vi "GUI Init - AOM.vi"(7 "Disabled":T1(ring), 8 "error in (no error)":errorcluster, 9 "Ch.names":string[](array[string]), 10 "Cluster":T3 {"Ch.value" min=-10.0 max=20.0 step=1.0 format="%.3g"}, 11 "GUI Refs":T2) -> (0 "error out":errorcluster, 2 "Data":dbl[](array[numeric]), 3 "reference out":refnum<vi>)   [LabVIEW 2017]
doc: "Initialize array's size and values for AOM Array by reference"
uses:
  Controls/AOM_GUI_Cluster.ctl
  Controls/GUI Referencies.ctl
  Controls/TDMS_GUI_Cluster.ctl
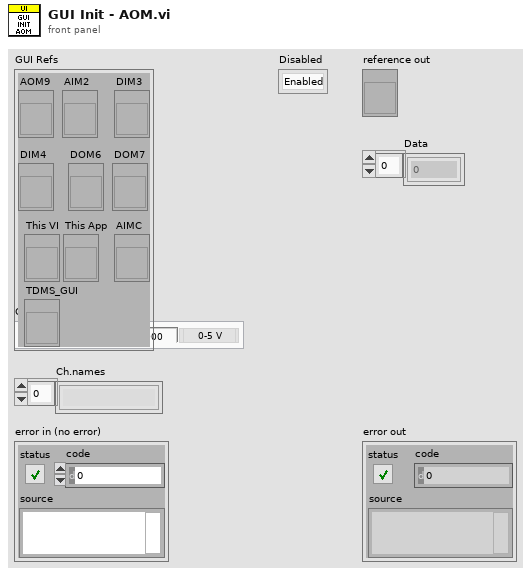
[diagram p1: front panel]
types:
  T1 = enum8{"Enabled", "Disabled", "Disabled and Grayed Out"}
  T2 = typedef "GUI Referencies.ctl" = cluster{"This VI":refnum<vi>, "This App":refnum<vi>, "DIM3":refnum<vi>, "DIM4":refnum<vi>, "DOM6":refnum<vi>, "DOM7":refnum<vi>, "AOM9":refnum<vi>, "AIM2":refnum<vi>, "AIMC":refnum<vi>, "TDMS_GUI":refnum<vi>}
  T3 = typedef "AOM_GUI_Cluster.ctl" = cluster{"Ch.name":string, "Ch.value":dbl, "Ch.mode":enum16{"0-5 V", "+/-10 V", "0-5 mA", "4-20 mA"}, "Num":string}
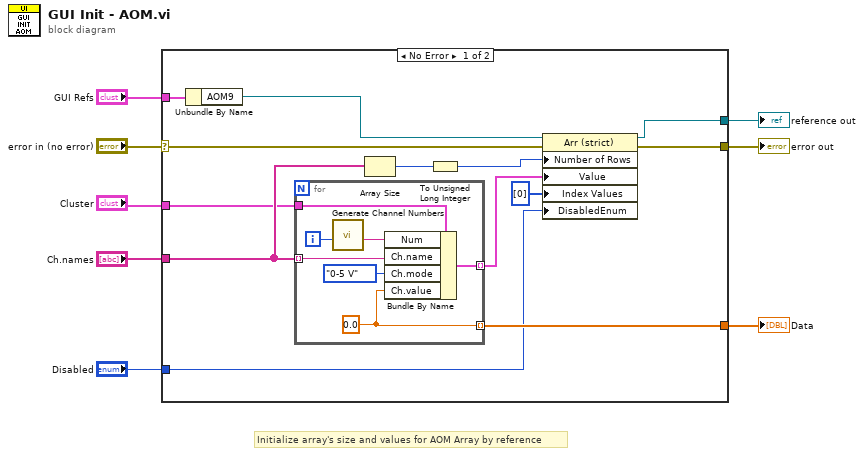
[diagram p0: block diagram]
diagram:
  # "Initialize array's size and values for AOM Array by reference"
  n1 = case shown="No Error" "error in (no error)" {
    selector: "error in (no error)" -> [w16 w29]
    tunnel: [w15 w29] -> w7
    tunnel: "Ch.names" -> [w18 _]
    tunnel: "GUI Refs" -> [w12 _]
    tunnel: "Cluster" -> [w17 _]
    tunnel: [w14 _] -> w4
    tunnel: [w10 _] -> w2
    tunnel: "Disabled" -> [w9 _]
    frame No Error {
      n2 = Unbundle By Name(w12) -> ("AOM9"=w11:refnum<vi>)
      n3 = for {
        tunnel: [w28] -> w14 mode=indexing
        tunnel: [w27] -> w13 mode=indexing
        tunnel: w18 -> [w26] mode=indexing
        tunnel: w17 -> [w25]
        i -> [w22]
        w28 = 0.0 ("Ch.value")
        n4 = call "Generate Channel Numbers.vi"("Index"=w22) -> ("Number"=w23:string)  [unwired: 9 in, 1 out]
        n5 = Bundle By Name(cluster=w25, "Num"=w23, "Ch.name"=w26, "Ch.mode"=enum16{"0-5 V", "+/-10 V", "0-5 mA", "4-20 mA"}."0-5 V", "Ch.value"=w28) -> (w27:T3)
      }
      n6 = Array Size(array=w18) -> (size(s)=w20:i32)
      n7 = To Unsigned Long Integer(number=w20) -> (unsigned 32bit integer=w19:u32)
      n8 = property class="Arr (strict)"(reference=w11, error in=w16, "Number of Rows"=w19, "Value"=w13, "Index Values"=u32[] [0], "DisabledEnum"=w9) -> (reference out=w10:refnum<vi>, error out=w15:errorcluster)
    }
    frame Error {
    }
  }
  "error out" <- w7
  "Data" <- w4
  "reference out" <- w2
